vi "Set Attenuation.vi"(0 "VISA Tegam1":refnum<visa-resource-name>="PXI4::12::INSTR", 5 "VISA Tegam2":refnum<visa-resource-name>="PXI4::14::INSTR", 7 "vertical range":dbl, 11 "error in":errorcluster) -> (4 "Requested Range":dbl, 6 "Gain Multiplier":dbl, 15 "error out":errorcluster)   [LabVIEW 2010]
uses:
  Tegam4040_Offset_Global.vi
  <instrlib>/Tegam4040/Tegam4040.lvlib
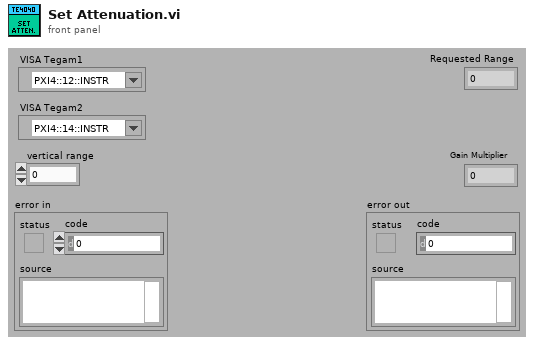
[diagram p1: front panel]
types:
  T1 = enum16{"Disable Calibration", "Enable Calibration"}
  T2 = enum16{"Attenuator Stage open", "Attenuation of 1", "Attenuation of 10", "Attenuation of 100"}
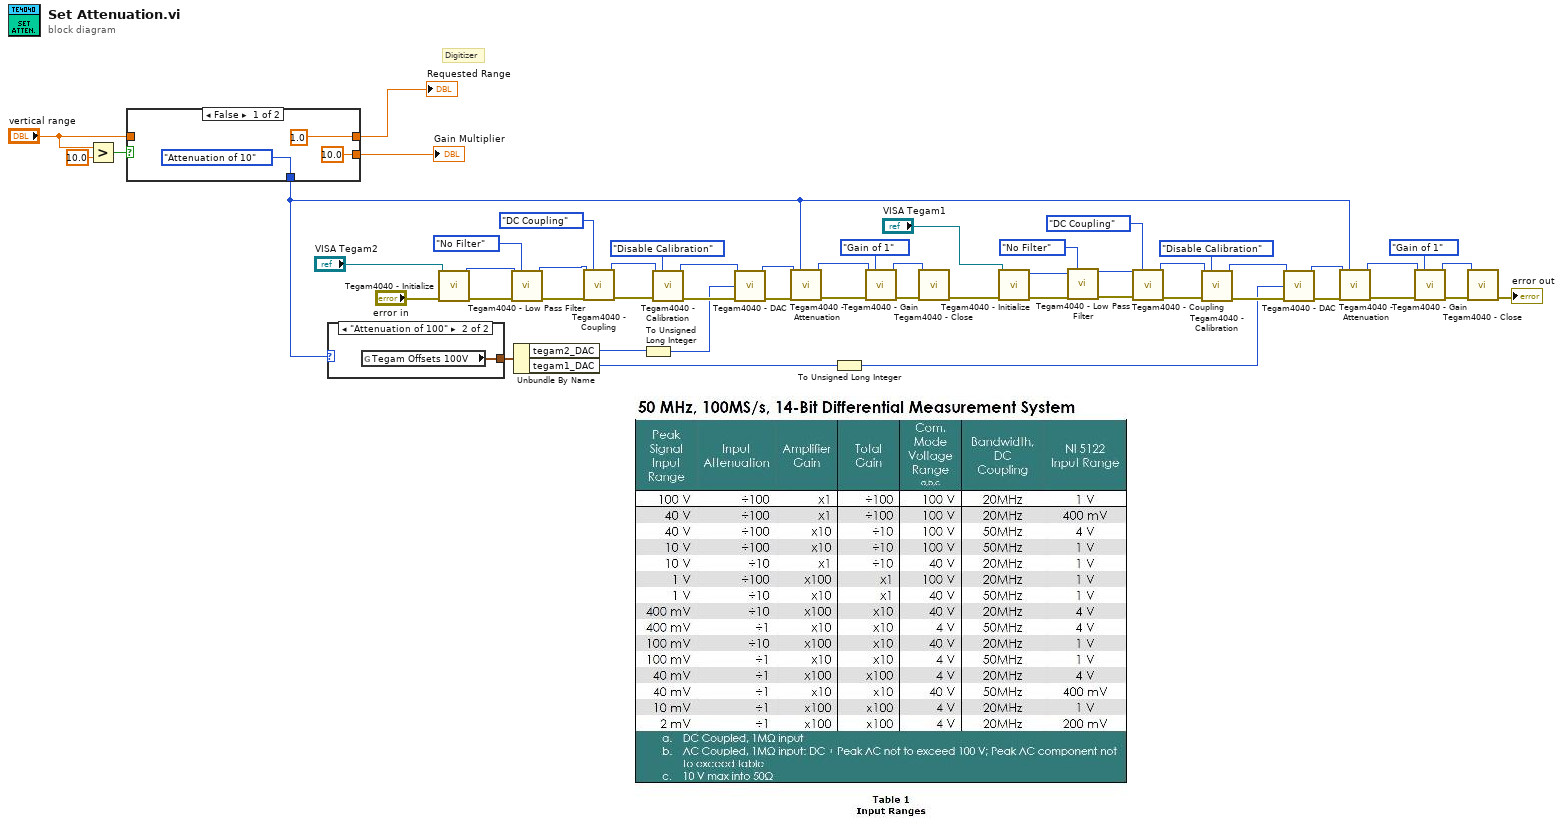
[diagram p0: block diagram]
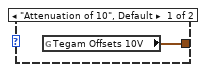
[diagram p2: hidden frame]
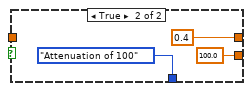
[diagram p3: hidden frame]
diagram:
  # "Digitizer"
  n1 = Greater?(x="vertical range", y=10.0) -> (0:w48:bool)
  n2 = case shown="False" w48 {
    tunnel: [T2."Attenuation of 10" ("Attenuation") T2."Attenuation of 100" ("Attenuation")] -> w15
    tunnel: [10.0 ("y") 100.0 ("y")] -> w51
    tunnel: [1.0 ("vertical range") 0.4 ("vertical range")] -> w50
    tunnel: "vertical range" -> [_ _]
    frame False {
    }
    frame True {
    }
  }
  "Gain Multiplier" <- w51
  "Requested Range" <- w50
  n3 = case shown="\"Attenuation of 100\"" w15 {
    tunnel: [w59 w60] -> w14
    frame "Attenuation of 10", Default {
      n4 = global read "Tegam4040_Offset_Global.vi" "Tegam Offsets 10V"() -> (w59:cluster{"tegam2_DAC":u16, "tegam1_DAC":u16})
    }
    frame "Attenuation of 100" {
      n5 = global read "Tegam4040_Offset_Global.vi" "Tegam Offsets 100V"() -> (w60:cluster{"tegam2_DAC":u16, "tegam1_DAC":u16})
    }
  }
  n6 = call <instrlib>:"Tegam4040 - Initialize.vi"("error in (no error)"="error in", "VISA Tegam4040"="VISA Tegam2") -> ("error out"=w13:errorcluster, "Instrument Session Handle"=w11:u32)  [unwired: 8 in]
  n7 = call <instrlib>:"Tegam4040 - Low Pass Filter.vi"("Instrument Session Handle In"=w11, "LP Filter"=enum16{"No Filter", "100kHz", "1MHz"}."No Filter", "error in (no error)"=w13) -> ("Instrument Session Handle Out (dupl)"=w10:u32, "error out"=w12:errorcluster)  [unwired: 11 in]
  n8 = Unbundle By Name(w14) -> ("tegam2_DAC"=w2:u16, "tegam1_DAC"=w16:u16)
  n9 = call <instrlib>:"Tegam4040 - Coupling.vi"("Instrument Session Handle In"=w10, "Coupling"=enum16{"DC Coupling", "AC Coupling"}."DC Coupling", "error in (no error)"=w12) -> ("Instrument Session Handle Out (dupl)"=w36:u32, "error out"=w35:errorcluster)  [unwired: 11 in]
  n10 = To Unsigned Long Integer(number=w2) -> (unsigned 32bit integer=w3:u32)
  n11 = call <instrlib>:"Tegam4040 - Calibration.vi"("Instrument Session Handle In"=w36, "Calibration"=T1."Disable Calibration", "error in (no error)"=w35) -> ("Instrument Session Handle Out (dupl)"=w39:u32, "error out"=w38:errorcluster)  [unwired: 11 in]
  n12 = call <instrlib>:"Tegam4040 - DAC.vi"("Instrument Session Handle In"=w39, "DAC"=w3, "error in (no error)"=w38) -> ("Instrument Session Handle Out (dupl)"=w34:u32, "error out"=w33:errorcluster)  [unwired: 11 in]
  n13 = call <instrlib>:"Tegam4040 - Attenuation.vi"("Instrument Session Handle In"=w34, "Attenuation"=w15, "error in (no error)"=w33) -> ("Instrument Session Handle Out (dupl)"=w45:u32, "error out"=w44:errorcluster)  [unwired: 11 in]
  n14 = To Unsigned Long Integer(number=w16) -> (unsigned 32bit integer=w1:u32)
  n15 = call <instrlib>:"Tegam4040 - Gain.vi"("Instrument Session Handle In"=w45, "Gain"=enum16{"Gain of 1", "Gain of 10", "Gain of 100"}."Gain of 1", "error in (no error)"=w44) -> ("Instrument Session Handle Out (dupl)"=w43:u32, "error out"=w42:errorcluster)  [unwired: 11 in]
  n16 = call <instrlib>:"Tegam4040 - Close.vi"("error in (no error)"=w42, "Instrument Session Handle"=w43) -> ("error out"=w19:errorcluster)  [unwired: 9 in]
  n17 = call <instrlib>:"Tegam4040 - Initialize.vi"("error in (no error)"=w19, "VISA Tegam4040"="VISA Tegam1") -> ("error out"=w8:errorcluster, "Instrument Session Handle"=w6:u32)  [unwired: 8 in]
  n18 = call <instrlib>:"Tegam4040 - Low Pass Filter.vi"("Instrument Session Handle In"=w6, "LP Filter"=enum16{"No Filter", "100kHz", "1MHz"}."No Filter", "error in (no error)"=w8) -> ("Instrument Session Handle Out (dupl)"=w5:u32, "error out"=w7:errorcluster)  [unwired: 11 in]
  n19 = call <instrlib>:"Tegam4040 - Coupling.vi"("Instrument Session Handle In"=w5, "Coupling"=enum16{"DC Coupling", "AC Coupling"}."DC Coupling", "error in (no error)"=w7) -> ("Instrument Session Handle Out (dupl)"=w23:u32, "error out"=w22:errorcluster)  [unwired: 11 in]
  n20 = call <instrlib>:"Tegam4040 - Calibration.vi"("Instrument Session Handle In"=w23, "Calibration"=T1."Disable Calibration", "error in (no error)"=w22) -> ("Instrument Session Handle Out (dupl)"=w26:u32, "error out"=w25:errorcluster)  [unwired: 11 in]
  n21 = call <instrlib>:"Tegam4040 - DAC.vi"("Instrument Session Handle In"=w26, "DAC"=w1, "error in (no error)"=w25) -> ("Instrument Session Handle Out (dupl)"=w21:u32, "error out"=w20:errorcluster)  [unwired: 11 in]
  n22 = call <instrlib>:"Tegam4040 - Attenuation.vi"("Instrument Session Handle In"=w21, "Attenuation"=w15, "error in (no error)"=w20) -> ("Instrument Session Handle Out (dupl)"=w32:u32, "error out"=w31:errorcluster)  [unwired: 11 in]
  n23 = call <instrlib>:"Tegam4040 - Gain.vi"("Instrument Session Handle In"=w32, "Gain"=enum16{"Gain of 1", "Gain of 10", "Gain of 100"}."Gain of 1", "error in (no error)"=w31) -> ("Instrument Session Handle Out (dupl)"=w30:u32, "error out"=w29:errorcluster)  [unwired: 11 in]
  n24 = call <instrlib>:"Tegam4040 - Close.vi"("error in (no error)"=w29, "Instrument Session Handle"=w30) -> ("error out"=→"error out":errorcluster)  [unwired: 9 in]
